vi "PSVCH_Config.vi"(8 "Error In (no error)":errorcluster, 9 "Var Info":T1, 10 "Formula[]":string[](array[string]), 11 "Tag[]":string[](array[string])) -> (0 "Error Out":errorcluster, 3 "Invalid":T2(array[cluster]))   [LabVIEW 2016]
panel:
  # "Data Out"
  # "Data In"
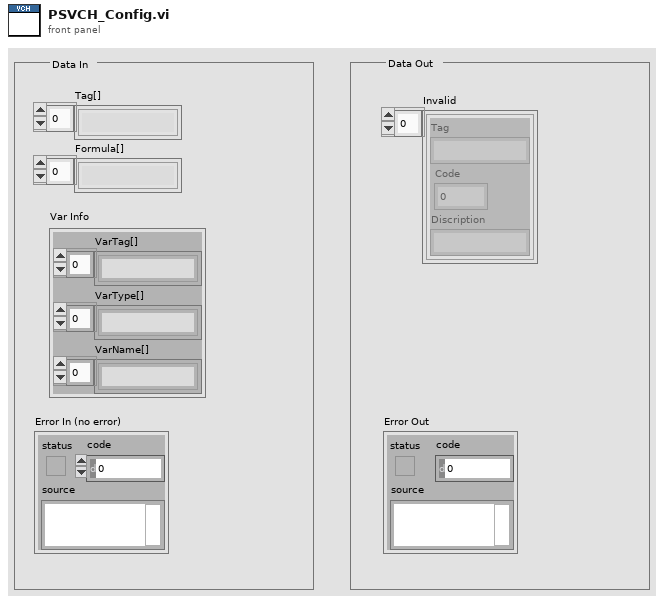
[diagram p1: front panel]
types:
  T1 = cluster{"VarTag[]":string[], "VarType[]":string[], "VarName[]":string[]}
  T2 = cluster{"Tag":string, "Code":i32, "Discription":string}[]
  T3 = cluster{"字符串":string, "Code":i32, "Discription":string}[]
  T4 = cluster{"字符串":string, "code":i32, "source":string}
  T5 = cluster{"字符串":string, "code":i32, "source":string}[]
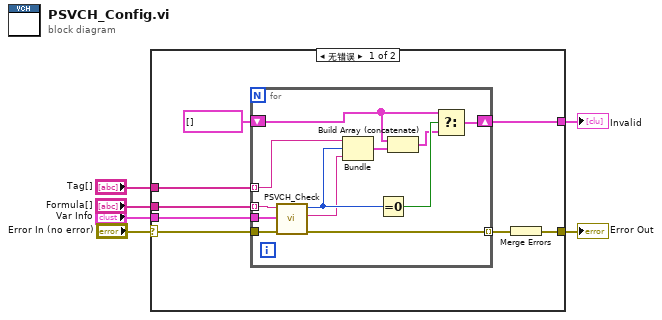
[diagram p0: block diagram]
diagram:
  n1 = case shown="无错误" "Error In (no error)" {
    selector: "Error In (no error)" -> [w13 w27]
    tunnel: [w11 w27] -> w5
    tunnel: [w12 _] -> w4
    tunnel: "Tag[]" -> [w9 _]
    tunnel: "Formula[]" -> [w8 _]
    tunnel: "Var Info" -> [w7 _]
    frame No Error {
      n2 = for {
        tunnel: w9 -> [w26] mode=indexing
        tunnel: w8 -> [w19] mode=indexing
        tunnel: w13 -> [w20]
        shift-right: [w23] -> w12
        shift-left: T3 [] -> [w22]
        tunnel: [w18] -> w10 mode=indexing
        tunnel: w7 -> [w15]
        n3 = call "PSVCH_Check.vi"("Error In (no error)"=w20, "VarList"=w15, "Formula"=w19) -> ("Error Out"=w18:errorcluster, "source"=w16:string, "code"=w17:i32)  [unwired: 6 in]
        n4 = Bundle("字符串"=w26, "code"=w17, "source"=w16) -> (w24:T4)  [unwired: 1 in]
        n5 = Equal To 0?(x=w17) -> (x = 0?=w25:bool)
        n6 = Build Array (concatenate)(w22, w24) -> (w21:T5)
        n7 = Select(t=w22, s=w25, f=w21) -> (s? t:f=w23:T5)
      }
      n8 = Merge Errors(w10) -> (w11:errorcluster)
    }
    frame Error {
    }
  }
  "Error Out" <- w5
  "Invalid" <- w4
